vi "EncoderReset.vi"(10 "EncoderDevRef 2":T1, 11 "EncoderDevRef":T1) -> ()   [LabVIEW 2015]
uses:
  <vilib>/Rock Robotics/WPI/Encoder/WPI_EncoderDevRef.ctl
  <vilib>/Rock Robotics/SystemInterfaces/Encoder/FPGA_EncoderIdx.ctl
  <vilib>/Rock Robotics/SystemInterfaces/Counter/FPGA_CounterCtrSystemIndex.ctl
  <vilib>/Rock Robotics/WPI/Encoder/WPI_EncoderType.ctl
  <vilib>/Rock Robotics/Network Tables/NT Read Boolean.vi
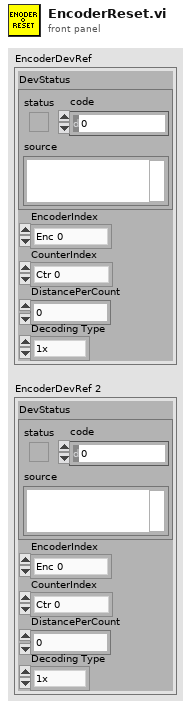
[diagram p1: front panel]
types:
  T1 = typedef "WPI_EncoderDevRef.ctl" = cluster{"DevStatus":errorcluster, "EncoderIndex":T2, "CounterIndex":T3, "DistancePerCount":dbl, "Decoding Type":T4}
  T2 = typedef "FPGA_EncoderIdx.ctl" = enum8{"Enc 0", "Enc 1", "Enc 2", "Enc 3", "Enc 4", "Enc 5", "Enc 6", "Enc 7", "Invalid"}
  T3 = typedef "FPGA_CounterCtrSystemIndex.ctl" = enum8{"Ctr 0", "Ctr 1", "Ctr 2", "Ctr 3", "Ctr 4", "Ctr 5", "Ctr 6", "Ctr 7", "Invalid"}
  T4 = typedef "WPI_EncoderType.ctl" = enum16{"1x", "2x", "4x"}
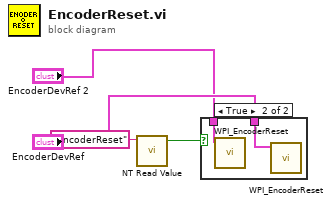
[diagram p0: block diagram]
diagram:
  n1 = call-poly <vilib>:"NT Read Value.vi"("Name"="EncoderReset") -> ("Boolean"=w1:bool)  [unwired: 9 in, 1 out]
  n2 = case shown="True" w1 {
    tunnel: "EncoderDevRef 2" -> [_ w6]
    tunnel: "EncoderDevRef" -> [_ w5]
    frame False {
    }
    frame True {
      n3 = call <vilib>:"WPI_EncoderReset.vi"("EncoderDevRef"=w6) -> ()  [unwired: 9 in, 2 out]
      n4 = call <vilib>:"WPI_EncoderReset.vi"("EncoderDevRef"=w5) -> ()  [unwired: 9 in, 2 out]
    }
  }
